vi "TM Head and Tail.vi"(11 "List":string[](array[string])) -> (2 "Tail List":string[](array[string]), 3 "Head":string)   [LabVIEW 2020, in "Tree Map.lvlib"]
doc: "Head - Return the first element, head of the input list. \nTail List - Drops the first element in the list and returns the rest. \nAdapts to wired data types."
uses:
  Tree Map.lvlib
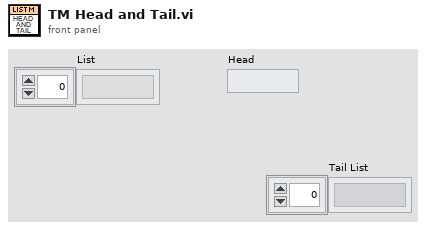
[diagram p1: front panel]
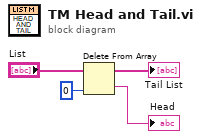
[diagram p0: block diagram]
diagram:
  n1 = Delete From Array(array="List", index=0) -> (deleted portion=→"Head":string, array with subset deleted=→"Tail List":string[])  [unwired: 1 in]
